vi "Read.vi"(8 "error in (no error)":errorcluster, 11 "TCP_Client in":refnum<class "TCP_Client.lvclass">) -> (0 "error out":errorcluster, 2 "Message":string, 3 "TCP_Client out":refnum<class "TCP_Client.lvclass">)   [LabVIEW 2018, in "TCP_Client.lvlib" / "TCP_Client.lvclass"]
uses:
  TCP_Client.lvclass
  TCP_Client.lvclass/TCP_Client.ctl
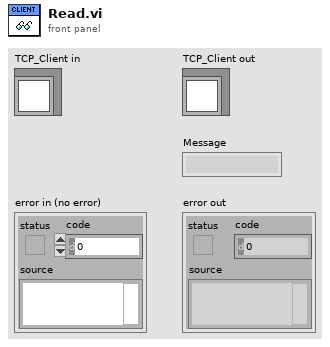
[diagram p1: front panel]
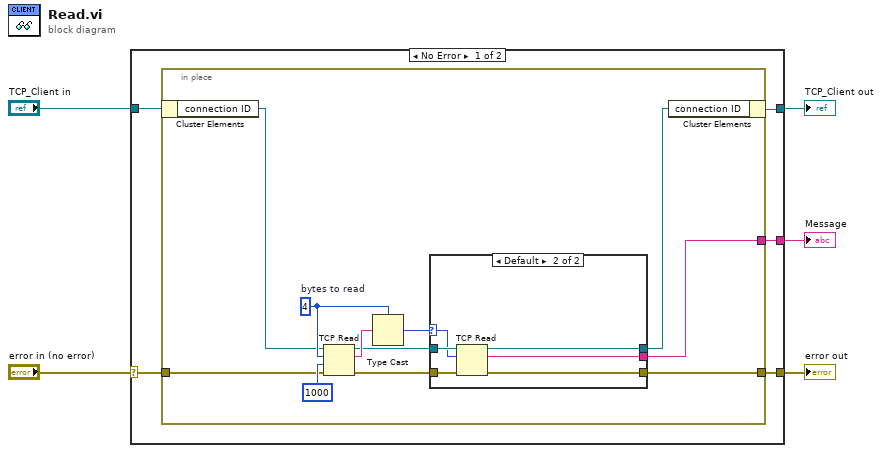
[diagram p0: block diagram]
diagram:
  n1 = case shown="No Error" "error in (no error)" {
    selector: "error in (no error)" -> [w10 w31]
    tunnel: [w9 w31] -> w4
    tunnel: [w7 w30] -> w2
    tunnel: "TCP_Client in" -> [w8 w30]
    tunnel: [w6 _] -> w1
    frame No Error {
      n2 = in-place {
        in-place-border: w10 -> [w15]
        in-place-border: [w14] -> w9
        in-place-border: [w11] -> w6
        w18 = 4  # bytes to read
        n3 = in-place-cluster #1(w8) -> ("connection ID"=w13:refnum<k5>)
        n4 = TCP Read(connection ID=w13, bytes to read=w18, error in (no error)=w15, 9:1000 ("timeout ms (25000)")) -> (connection ID out=w20:refnum<k5>, data out=w21:string, error out=w19:errorcluster)  [unwired: 1 in]
        n5 = Type Cast(type=w18, x=w21) -> (*(type *) &x=w17:i32)
        n6 = case shown="Default" w17 {
          selector: w17 -> [_ w25]
          tunnel: w20 -> [w23 w29]
          tunnel: w19 -> [w22 w28]
          tunnel: [w23 w27] -> w12
          tunnel: [w22 w26] -> w14
          tunnel: [_ w24] -> w11
          frame ..0 {
            # "The server has not written any data"
          }
          frame Default {
            n7 = TCP Read(connection ID=w29, bytes to read=w25, error in (no error)=w28) -> (connection ID out=w27:refnum<k5>, data out=w24:string, error out=w26:errorcluster)  [unwired: 2 in]
          }
        }
        n8 = in-place-cluster #1("connection ID"=w12) -> (w7:refnum<class "TCP_Client.lvclass">)
      }
    }
    frame Error {
    }
  }
  "error out" <- w4
  "TCP_Client out" <- w2
  "Message" <- w1
